vi "gratingToSALGrating.vi"(8 "error in (no error)":errorcluster, 9 "SALGrating in":enum16{"", "Blue", "Red", "Mirror"}(ring), 10 "MonochromatorGrating in":T1, 11 "MonoClientCommunicator in":refnum<class "MonoClientCommunicator.lvclass">) -> (0 "error out":errorcluster, 1 "MonochromatorGrating out":T1, 2 "SALGrating out":enum16{"", "Blue", "Red", "Mirror"}(ring), 3 "MonoClientCommunicator out":refnum<class "MonoClientCommunicator.lvclass">)   [LabVIEW 2016, in "MonoClientCommunicator.lvclass"]
uses:
  MonoClientCommunicator.lvclass
  Typedefs/GratingType.ctl
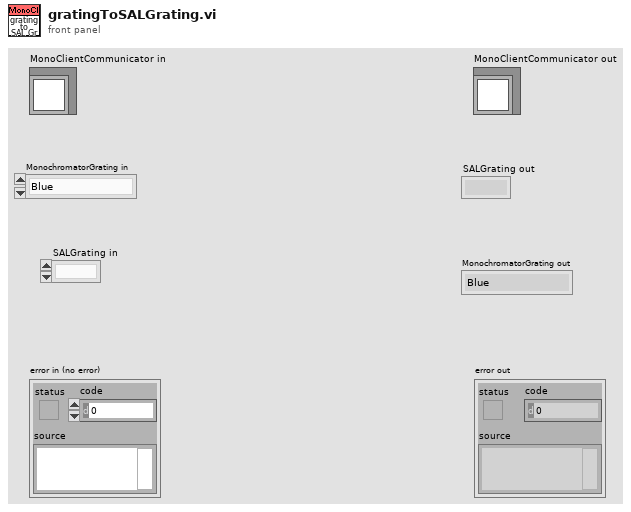
[diagram p1: front panel]
types:
  T1 = typedef "GratingType.ctl" = enum16{"Blue", "Red", "Mirror"}
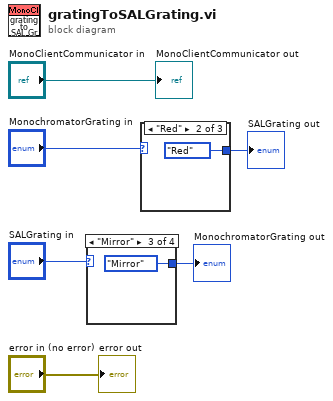
[diagram p0: block diagram]
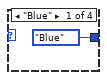
[diagram p2: hidden frame]
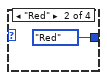
[diagram p3: hidden frame]
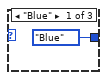
[diagram p5: hidden frame]
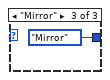
[diagram p6: hidden frame]
diagram:
  n1 = case shown="\"Mirror\"" "SALGrating in" {
    tunnel: [GratingType."Blue" ("MonochromatorGrating out") GratingType."Red" ("MonochromatorGrating out") GratingType."Mirror" ("MonochromatorGrating out") _] -> w2
    frame "Blue" {
    }
    frame "Red" {
    }
    frame "Mirror" {
    }
    frame "" {
    }
  }
  "MonochromatorGrating out" <- w2
  n2 = case shown="\"Red\"" "MonochromatorGrating in" {
    tunnel: [enum16{"", "Blue", "Red", "Mirror"}."Blue" ("SALGrating out") enum16{"", "Blue", "Red", "Mirror"}."Red" ("SALGrating out") enum16{"", "Blue", "Red", "Mirror"}."Mirror" ("SALGrating out")] -> w1
    frame "Blue" {
    }
    frame "Red" {
    }
    frame "Mirror" {
    }
  }
  "SALGrating out" <- w1
  "error out" <- "error in (no error)"
  "MonoClientCommunicator out" <- "MonoClientCommunicator in"
